vi "1Centigrados a F.vi"(2 "error in (no error)":errorcluster, 3 "Selector":bool, 4 "Temperatura":dbl) -> (0 "error out":errorcluster, 1 "Conversion":dbl)   [LabVIEW 2016]
doc: "Este VI es un convertidor de grados C a F y viceversa"
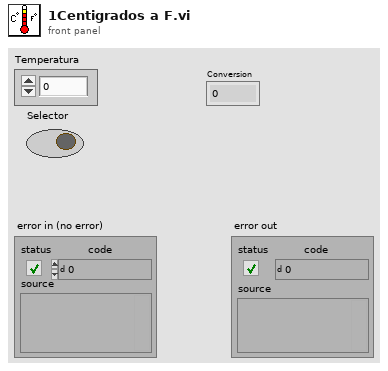
[diagram p1: front panel]
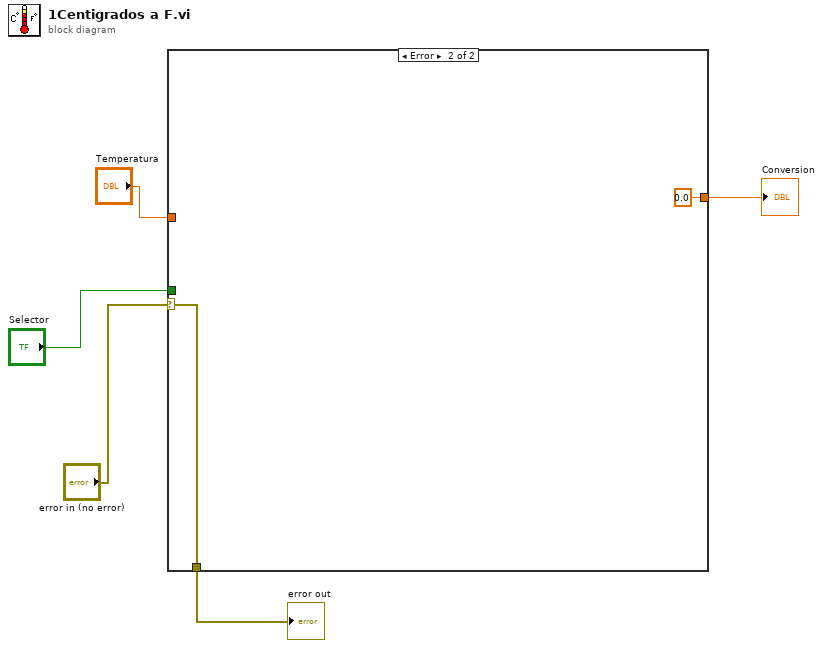
[diagram p0: block diagram]
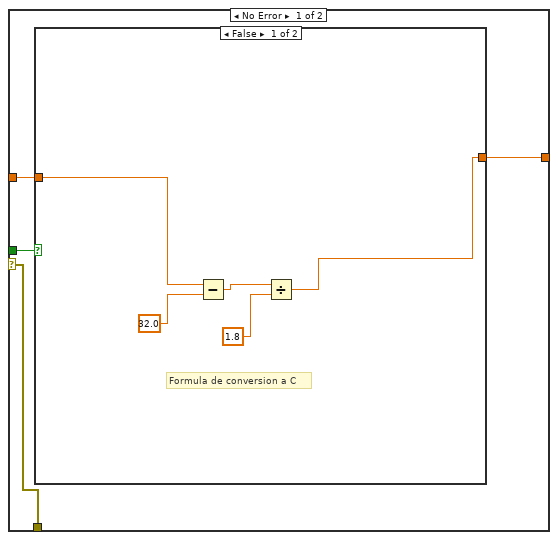
[diagram p2: hidden frame]
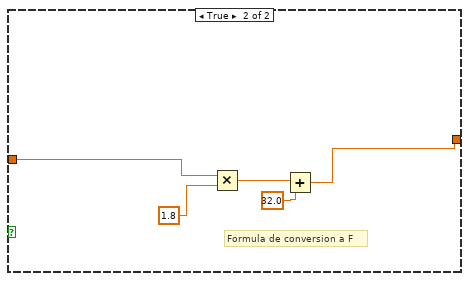
[diagram p3: hidden frame]
diagram:
  n1 = case shown="Error" "error in (no error)" {
    selector: "error in (no error)" -> [w6 w21]
    tunnel: "Selector" -> [w9 _]
    tunnel: "Temperatura" -> [w8 _]
    tunnel: [w7 0.0] -> w3
    tunnel: [w6 w21] -> w1
    frame No Error {
      n2 = case shown="False" w9 {
        tunnel: w8 -> [w11 w16]
        tunnel: [w10 w15] -> w7
        frame False {
          # "Formula de conversion a C"
          n3 = Subtract(x=w11, y=32.0) -> (x-y=w13:dbl)
          n4 = Divide(x=w13, y=1.8) -> (x/y=w10:dbl)
        }
        frame True {
          # "Formula de conversion a F"
          n5 = Multiply(x=w16, y=1.8) -> (x*y=w19:dbl)
          n6 = Add(x=w19, y=32.0) -> (x+y=w15:dbl)
        }
      }
    }
    frame Error {
    }
  }
  "Conversion" <- w3
  "error out" <- w1
